vi "Ultrasonic_Code_EV3.vi"() -> ()   [LabVIEW 2012]
uses:
  SubVIs/LVPresent_Globals.vi
panel:
  in  "Tab Control":enum32{"Page 1", "Page 2"}(tab)
  in  "Open":bool
  in  "Need a hint":bool
  in  "Ans. 6":bool
  in  "Ans. 5":bool
  in  "Ans. 4":bool
  in  "Back":bool
  # "Using the Ultrasonic Sensor\n\nNow, let's try using the Ultrasonic sensor. Add the sensor onto your robot, and then write a program in order to stop the robot 10 cm from the wall. Click the Open button to start a new VI. If you're stuck on how to add the sensor, check out the EV3 manual or the help! Also, for now it would probably be easier to leave on AutoTooling."
  # "Step 2:\n\nAfter you get the code running, try modifying your code so that the robot slows to half of its speed at 20 cm, and then stops fully at 10 cm."
  # "Extra Challenge:\n\nNow, try slowing the car proportionally, so that as the car nears 10 cm, it slows down gradually as it gets closer."
  # "Hint 1: Check out the functions under the Sensors tab  and the Timing  tab under Complete, I/O and MINDSTORMS Robotics. Remember that if you do not know what a function does, you can turn on Show Context Help, under the Help tab. \n\n\n\n\n\nHint 2: The Ultrasonic sensor works from a distance of 0-250 cm. Farther from that, the distance from an object is essentially infinity. \n\n\n\n\n\nHint 3: In order to get the object to stop 10 cm before the wall, you want to slow it at a speed of n - 10, where n is the distance from the wall. \n\n\n\n\n\nHelpful Tip: When creating a constant, you can simply right click on the terminal you wish to wire to, click create-->constant. Note that constants aren't always necessarily numbers."
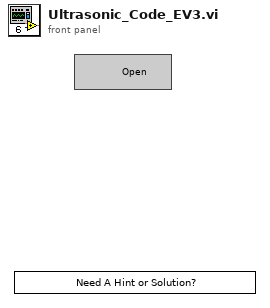
[diagram p1: front panel]
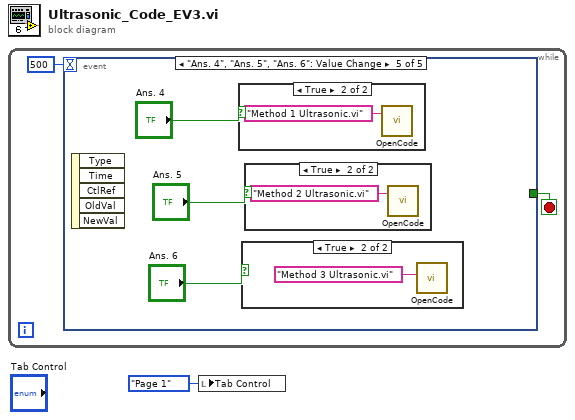
[diagram p0: block diagram]
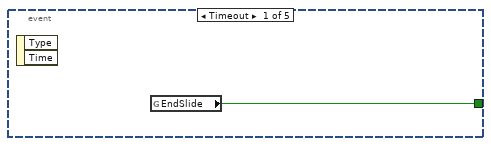
[diagram p2: hidden frame]
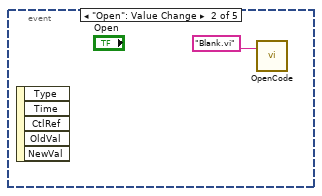
[diagram p3: hidden frame]
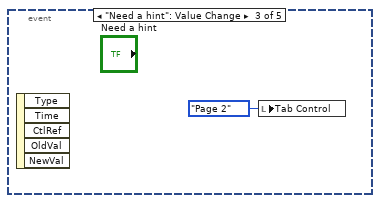
[diagram p4: hidden frame]
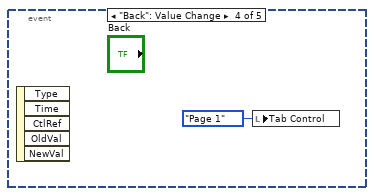
[diagram p5: hidden frame]
diagram:
  n1 = while {
    stop <- w3 stop-if-true
    n2 = event shown="[4] \"Ans. 4\", \"Ans. 5\", \"Ans. 6\": Value Change" {
      selector: _ -> [_ _ _ _ _]
      dyn-events: _ -> [_ _ _ _ _]
      timeout: 500 -> [_ _ _ _ _]
      tunnel: [w4 _ _ _ _] -> w3
      event Timeout {
        n3 = event-data() -> ()  [unwired: 1 in, 2 out]
        n4 = global read "LVPresent_Globals.vi" "EndSlide"() -> (w4:bool)
      }
      event "Open": Value Change {
        n5 = event-data() -> ()  [unwired: 1 in, 5 out]
        n6 = call "OpenCode.vi"("Code name"="Blank.vi") -> ()  [unwired: 3 in]
      }
      event "Need a hint": Value Change {
        n7 = event-data() -> ()  [unwired: 1 in, 5 out]
        n8 = local write "Tab Control"(enum32{"Page 1", "Page 2"}."Page 2" ("Tab Control")) -> ()
      }
      event "Back": Value Change {
        n9 = event-data() -> ()  [unwired: 1 in, 5 out]
        n10 = local write "Tab Control"(enum32{"Page 1", "Page 2"}."Page 1" ("Tab Control")) -> ()
      }
      event "Ans. 4", "Ans. 5", "Ans. 6": Value Change {
        n11 = event-data() -> ()  [unwired: 1 in, 5 out]
        n12 = case shown="True" "Ans. 4" {
          frame False {
          }
          frame True {
            n13 = call "OpenCode.vi"("Code name"="Method 1 Ultrasonic.vi") -> ()  [unwired: 3 in]
          }
        }
        n14 = case shown="True" "Ans. 6" {
          frame False {
          }
          frame True {
            n15 = call "OpenCode.vi"("Code name"="Method 3 Ultrasonic.vi") -> ()  [unwired: 3 in]
          }
        }
        n16 = case shown="True" "Ans. 5" {
          frame False {
          }
          frame True {
            n17 = call "OpenCode.vi"("Code name"="Method 2 Ultrasonic.vi") -> ()  [unwired: 3 in]
          }
        }
      }
    }
  }
  n18 = local write "Tab Control"(enum32{"Page 1", "Page 2"}."Page 1" ("Tab Control")) -> ()
